vi "Select Message Log Array.vi"(11 "Message Log in":refnum<class "Message Log.lvclass">) -> (1 "Selected Array":string[][](array[string]), 3 "Message Log out":refnum<class "Message Log.lvclass">)   [LabVIEW 2017, in "Message Log.lvclass"]
uses:
  Message Log.lvclass
  Message Log.lvclass/Message Log.ctl
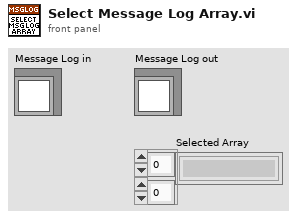
[diagram p1: front panel]
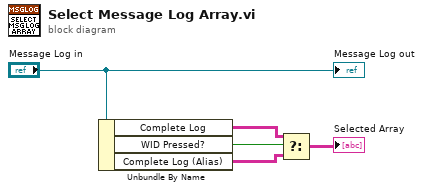
[diagram p0: block diagram]
diagram:
  n1 = Unbundle By Name("Message Log in") -> ("Complete Log"=w4:string[][], "WID Pressed?"=w2:bool, "Complete Log (Alias)"=w3:string[][])
  n2 = Select(t=w4, s=w2, f=w3) -> (s? t:f=→"Selected Array":string[][])
  "Message Log out" <- "Message Log in"
